vi "5-20-2015.vi"() -> ()   [LabVIEW 2014]
uses:
  <vilib>/rvi/Emulation/niFpgaGetClockAttributes.vi
  <vilib>/rvi/Emulation/niFpgaSctlEmulationGetInTimedLoop.vi
  <vilib>/rvi/Emulation/niFpgaEmulationReportErrorSimple.vi
  <vilib>/rvi/Emulation/niFpgaCriticalErrorInLSC.vi
  SPIBus0/IO Node Logic Template_SPIBus0.lvlib
panel:
  out "Received Data":u64
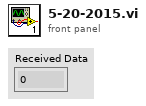
[diagram p1: front panel]
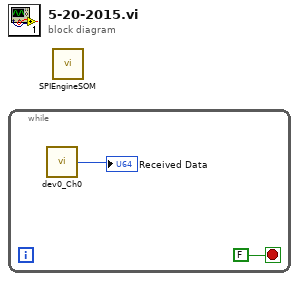
[diagram p0: block diagram]
diagram:
  n1 = while {
    stop <- FALSE stop-if-true
    n2 = call "dev0_Ch0.vi"() -> ("Received Data"=→"Received Data":u64)  [unwired: 15 in]
  }
  n3 = call "SPIEngineSOM.vi"() -> ()  [unwired: 12 in]
